vi "HtttpMethod1.vi"(7 "http":enum16{"open", "post", "close", "idle"}(ring), 8 "error constant":errorcluster, 10 "file":path, 11 "url":string) -> (0 "error out":errorcluster, 2 "body":string, 3 "headers":string)   [LabVIEW 2019]
uses:
  <vilib>/httpClient/MultipartData.ctl
  LLB/Message/Ctrl/MsgDataInput.ctl
  LLB/Message/Ctrl/MsgPageSelect.ctl
  LLB/Message/Ctrl/LogType.ctl
  <vilib>/httpClient/LabVIEWHTTPClient.lvlib
  LLB/Message/MsgShowAndLog.lvlib
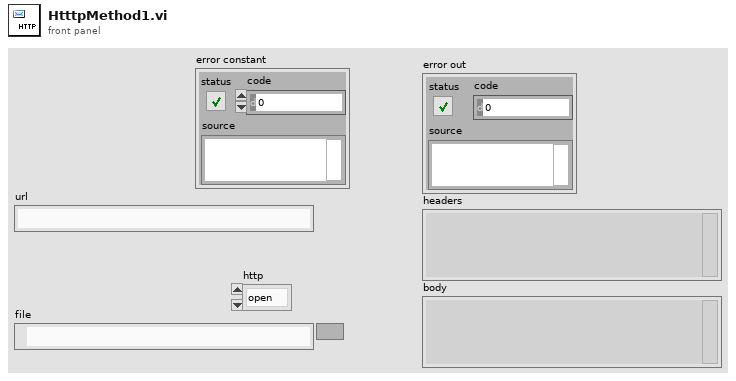
[diagram p1: front panel]
types:
  T1 = typedef "MsgDataInput.ctl" = cluster{"MsgPageSelect":T2, "LogType":T3, "Msg":string, "Time":string}
  T2 = typedef "MsgShowAndLog.lvlib/MsgPageSelect.ctl" = enum16{"System", "Comm", "IO", "Action", "Alarm"}
  T3 = typedef "MsgShowAndLog.lvlib/LogType.ctl" = enum16{"Auto", "Manual", "Handshake", "Error"}
  T4 = typedef "LabVIEWHTTPClient.lvlib/MultipartData.ctl" = cluster{"Name":string, "Value":string, "File":path, "Filename":string, "MIME type":string}
  T5 = typedef "LabVIEWHTTPClient.lvlib/ClientHandle.ctl" = refnum<k1>
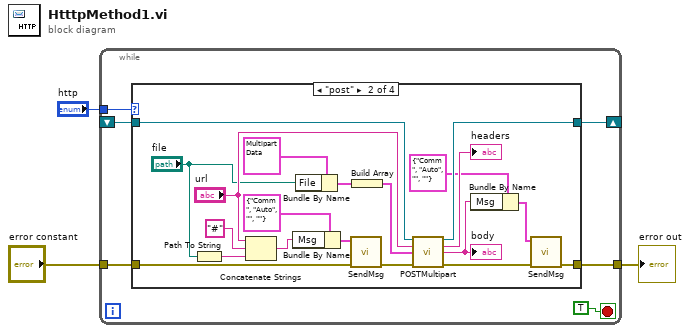
[diagram p0: block diagram]
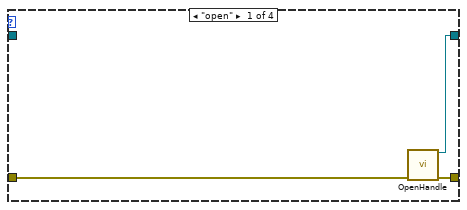
[diagram p2: hidden frame]
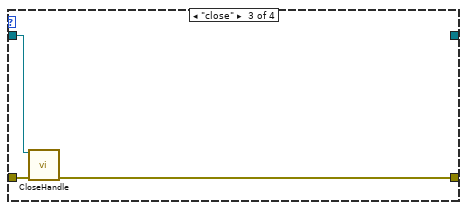
[diagram p3: hidden frame]
diagram:
  n1 = while {
    tunnel: "http" -> [w9]
    tunnel: [w7] -> w1
    tunnel: "error constant" -> [w6]
    shift-right: [w5] -> _
    shift-left: _ -> [w4]
    stop <- TRUE stop-if-true
    n2 = case shown="\"post\"" w9 {
      tunnel: [w12 w13 w34 w37] -> w7
      tunnel: w6 -> [w11 w18 w33 w37]
      tunnel: [w10 w31 _ w36] -> w5
      tunnel: w4 -> [_ w32 w35 w36]
      frame "open" {
        n3 = call <vilib>:"OpenHandle.vi"("error in (no error)"=w11) -> ("client handle out"=w10:T5, "error out"=w12:errorcluster)  [unwired: 13 in]
      }
      frame "post" {
        n4 = Path To String(path="file") -> (string=w21:string)
        n5 = Concatenate Strings("url", "#" ("string"), w21) -> (w26:string)
        n6 = Bundle By Name(cluster=T1 {"MsgPageSelect"=enum."Comm", "LogType"=enum."Auto", "Msg"="", "Time"=""} ("DataIn"), "Msg"=w26) -> (w25:T1)
        n7 = Bundle By Name(cluster=T4 {"Name"="file", "Value"="", "File"=path "", "Filename"="1.png", "MIME type"="image/png"} ("Element"), "File"="file") -> (w28:T4)
        n8 = call "SendMsg.vi"("error in (no error)"=w18, "DataIn"=w25) -> ("error out"=w19:errorcluster)  [unwired: 9 in]
        n9 = Build Array(w28) -> (w27:T4[])
        n10 = call <vilib>:"POSTMultipart.vi"("client handle"=w32, "url"="url", "data"=w27, "error in (no error)"=w19) -> ("client handle out"=w31:T5, "headers"=→"headers":string, "body"=w15:string, "error out"=w14:errorcluster)  [unwired: 8 in]
        "body" <- w15
        n11 = Bundle By Name(cluster=T1 {"MsgPageSelect"=enum."Comm", "LogType"=enum."Auto", "Msg"="", "Time"=""} ("DataIn"), "Msg"=w15) -> (w16:T1)
        n12 = call "SendMsg.vi"("error in (no error)"=w14, "DataIn"=w16) -> ("error out"=w13:errorcluster)  [unwired: 9 in]
      }
      frame "close" {
        n13 = call <vilib>:"CloseHandle.vi"("client handle"=w35, "error in (no error)"=w33) -> ("error out"=w34:errorcluster)  [unwired: 13 in]
      }
      frame "idle", Default {
      }
    }
  }
  "error out" <- w1
